vi "Make Comp.vi"(8 "error in (no error)":errorcluster, 11 "Setup File in":refnum<class "Setup File.lvclass">) -> (0 "error out":errorcluster, 3 "Setup File out":refnum<class "Setup File.lvclass">)   [LabVIEW 2018, in "Setup File.lvclass"]
doc: "Este VI cria um arquivo texto com a configuração para aquisição de imagens de comparação (configuração ainda não definida)"
uses:
  Setup File.lvclass
  Setup File.lvclass/Setup File.ctl
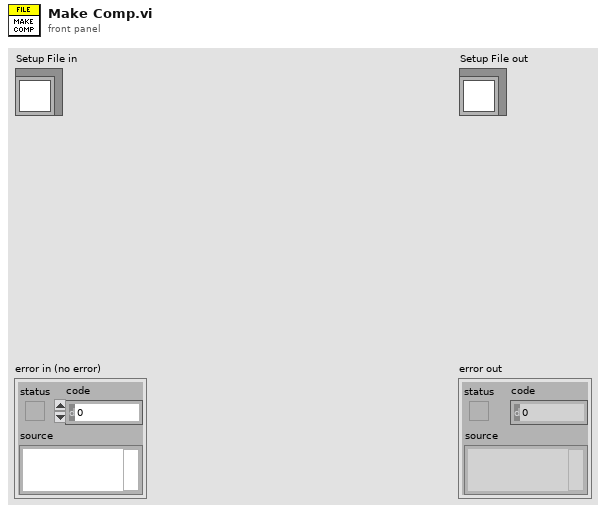
[diagram p1: front panel]
types:
  T1 = enum16{"open", "replace", "create", "open or create", "replace or create", "replace or create with confirmation"}
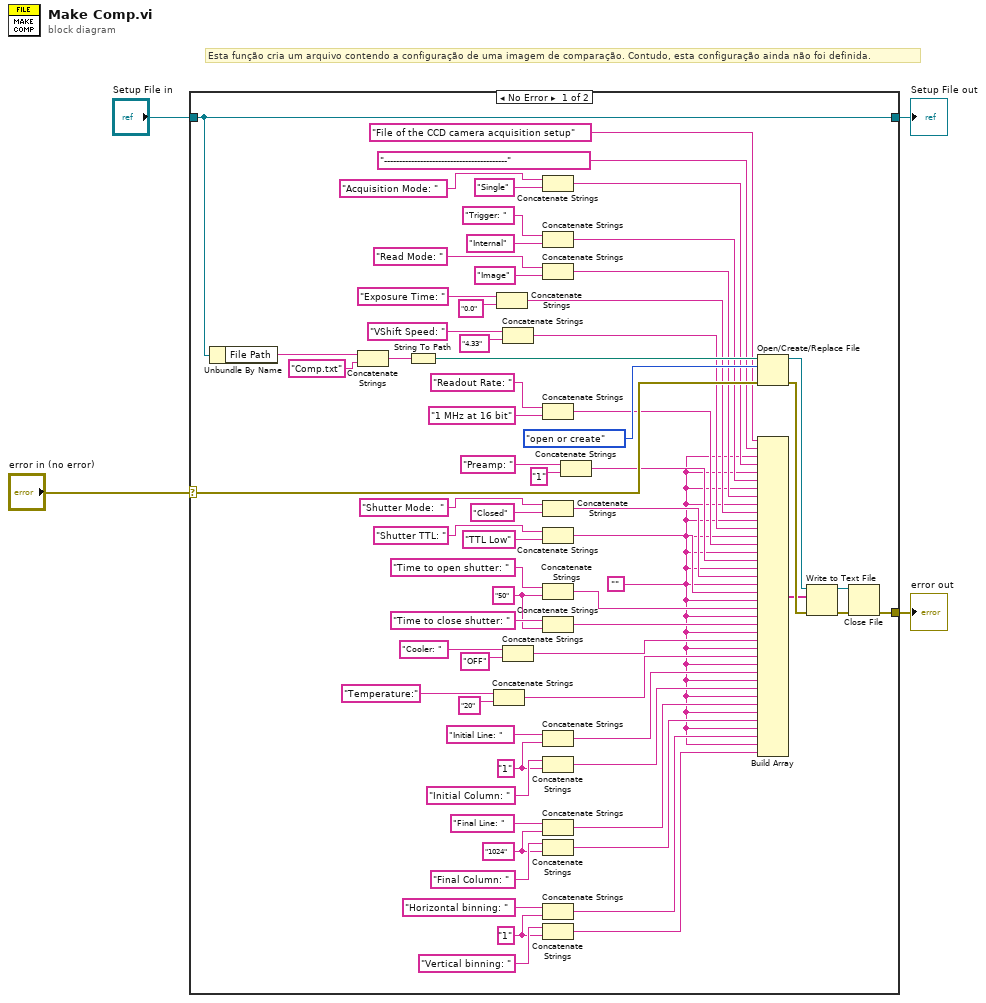
[diagram p0: block diagram]
diagram:
  # "Esta função cria um arquivo contendo a configuração de uma imagem de comparação. Contudo, esta configuração ainda não foi definida."
  n1 = case shown="No Error" "error in (no error)" {
    selector: "error in (no error)" -> [w73 w75]
    tunnel: [w70 w75] -> w2
    tunnel: [w67 w74] -> w3
    tunnel: "Setup File in" -> [w67 w74]
    frame No Error {
      w6 = "1"
      w7 = "1024"
      w8 = "1"
      w11 = "50"
      w22 = ""
      n2 = Unbundle By Name(w67) -> ("File Path"=w66:string)
      n3 = Concatenate Strings(w66, "Comp.txt") -> (w65:string)
      n4 = String To Path(string=w65) -> (path=w64:path)
      n5 = Concatenate Strings("Temperature:", "20") -> (w29:string)
      n6 = Concatenate Strings("Exposure Time: ", "0.0") -> (w38:string)
      n7 = Concatenate Strings("VShift Speed: ", "4.33") -> (w37:string)
      n8 = Concatenate Strings("Cooler: ", "OFF") -> (w30:string)
      n9 = Concatenate Strings("Acquisition Mode: ", "Single") -> (w41:string)
      n10 = Concatenate Strings("Trigger: ", "Internal") -> (w40:string)
      n11 = Concatenate Strings("Read Mode: ", "Image") -> (w39:string)
      n12 = Concatenate Strings("Readout Rate: ", "1 MHz at 16 bit") -> (w36:string)
      n13 = Concatenate Strings("Shutter Mode:  ", "Closed") -> (w34:string)
      n14 = Concatenate Strings("Shutter TTL: ", "TTL Low") -> (w33:string)
      n15 = Concatenate Strings("Time to open shutter: ", w11) -> (w32:string)
      n16 = Concatenate Strings("Time to close shutter: ", w11) -> (w31:string)
      n17 = Concatenate Strings("Initial Line: ", w8) -> (w28:string)
      n18 = Concatenate Strings("Initial Column: ", w8) -> (w27:string)
      n19 = Concatenate Strings("Final Line: ", w7) -> (w26:string)
      n20 = Concatenate Strings("Final Column: ", w7) -> (w25:string)
      n21 = Concatenate Strings("Horizontal binning: ", w6) -> (w24:string)
      n22 = Concatenate Strings("Vertical binning: ", w6) -> (w23:string)
      n23 = Concatenate Strings("Preamp: ", "1") -> (w35:string)
      n24 = Open/Create/Replace File(file path (use dialog)=w64, error in=w73, operation (0:open)=T1."open or create") -> (refnum out=w69:refnum<file>, error out=w72:errorcluster)  [unwired: 3 in, 1 out]
      n25 = Build Array("File of the CCD camera acquisition setup" ("string"), "-----------------------------------------" ("string"), w22, w41, w22, w40, w22, w39, w22, w38, w22, w37, w22, w36, w22, w35, w22, w34, w22, w33, w22, w32, w22, w31, w22, w30, w22, w29, w22, w28, w22, w27, w22, w26, w22, w25, w22, w24, w22, w23) -> (w21:string[])
      n26 = Write to Text File(file (use dialog)=w69, text=w21, error in=w72) -> (refnum out=w68:refnum<file>, error out=w71:errorcluster)  [unwired: 1 in, 1 out]
      n27 = Close File(refnum=w68, error in=w71) -> (error out=w70:errorcluster)  [unwired: 1 out]
    }
    frame Error {
    }
  }
  "error out" <- w2
  "Setup File out" <- w3
